vi "projector check.vi"() -> ()   [LabVIEW 2019]
uses:
  Setting Lib.lvlib
panel:
  out "Projector Status 26":bool
  out "Projector Status 30":bool
  out "Projector Status 29":bool
  out "Projector Status 27":bool
  out "Projector Status 28":bool
  out "error out 7":errorcluster
  in  "Threshold 26":dbl=0.01 format="%#_13g"
  in  "Threshold 30":dbl=0.01 format="%#_13g"
  in  "Threshold 29":dbl=0.01 format="%#_13g"
  in  "Threshold 27":dbl=0.01 format="%#_13g"
  in  "Threshold 28":dbl=0.01 format="%#_13g"
  out "error out 6":errorcluster
  out "error out 5":errorcluster
  out "error out 4":errorcluster
  out "error out 3":errorcluster
  out "error out 2":errorcluster
  out "error out":errorcluster
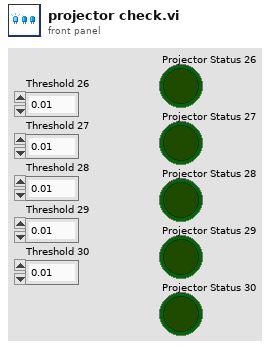
[diagram p1: front panel]
types:
  T1 = typedef "IMAQ Image.ctl" = refnum<image>
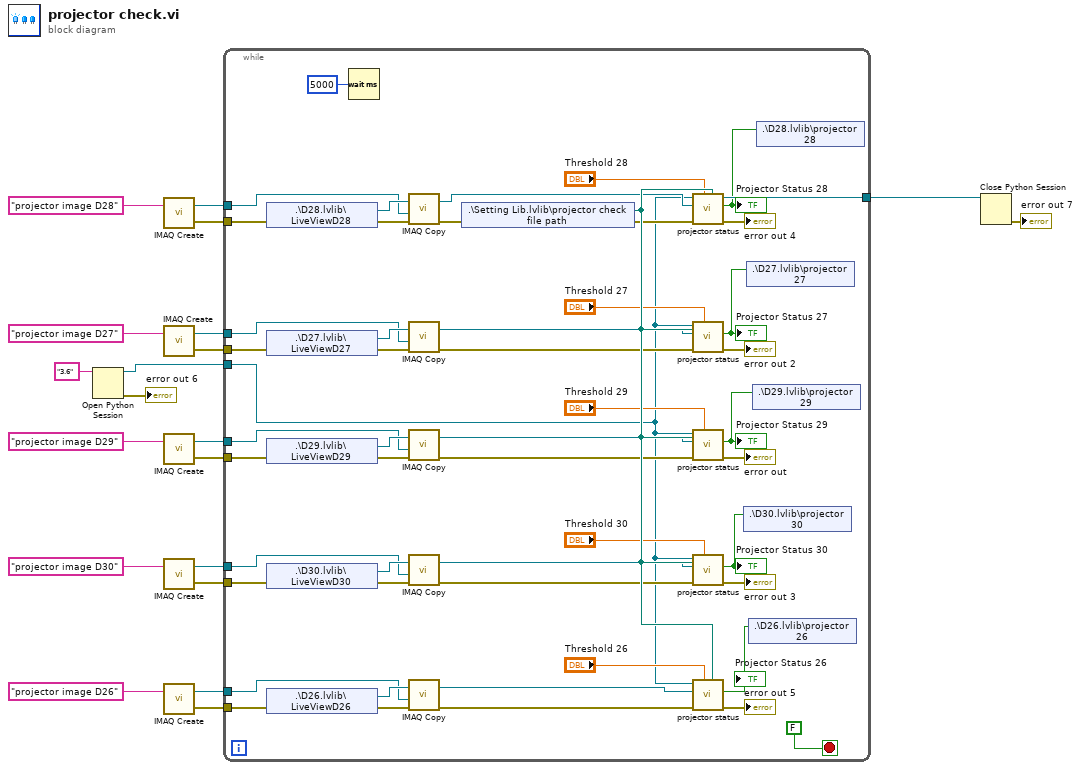
[diagram p0: block diagram]
diagram:
  n1 = Open Python Session(python version="3.6" ("Python version")) -> (session out=w3:refnum<k35>, error out=→"error out 6":errorcluster)  [unwired: 2 in]
  n2 = call "IMAQ Create"("Image Name"="projector image D28") -> ("New Image"=w11:T1, "error out"=w10:errorcluster)  [unwired: 4 in]
  n3 = call "IMAQ Create"("Image Name"="projector image D27") -> ("New Image"=w13:T1, "error out"=w12:errorcluster)  [unwired: 4 in]
  n4 = call "IMAQ Create"("Image Name"="projector image D29") -> ("New Image"=w9:T1, "error out"=w8:errorcluster)  [unwired: 4 in]
  n5 = call "IMAQ Create"("Image Name"="projector image D30") -> ("New Image"=w7:T1, "error out"=w6:errorcluster)  [unwired: 4 in]
  n6 = call "IMAQ Create"("Image Name"="projector image D26") -> ("New Image"=w15:T1, "error out"=w14:errorcluster)  [unwired: 4 in]
  n7 = while {
    tunnel: w15 -> [w66]
    tunnel: w14 -> [w65]
    tunnel: w13 -> [w58]
    tunnel: w12 -> [w57]
    tunnel: w11 -> [w52]
    tunnel: w10 -> [w51]
    tunnel: w9 -> [w45]
    tunnel: w8 -> [w44]
    tunnel: w7 -> [w38]
    tunnel: w6 -> [w37]
    tunnel: w3 -> [w28]
    tunnel: [w26] -> w2
    stop <- FALSE stop-if-true
    n8 = shared-variable ".\\D28.lvlib\\LiveViewD28"(error in=w51) -> (w54:refnum<image>, error out=w55:errorcluster)
    n9 = shared-variable ".\\D27.lvlib\\LiveViewD27"(error in=w57) -> (w62:refnum<image>, error out=w61:errorcluster)
    n10 = shared-variable ".\\D29.lvlib\\LiveViewD29"(error in=w44) -> (w49:refnum<image>, error out=w48:errorcluster)
    n11 = shared-variable ".\\D30.lvlib\\LiveViewD30"(error in=w37) -> (w41:refnum<image>, error out=w39:errorcluster)
    n12 = shared-variable ".\\D26.lvlib\\LiveViewD26"(error in=w65) -> (w70:refnum<image>, error out=w68:errorcluster)
    n13 = Wait (ms)(milliseconds to wait=u32 5000) -> ()  [unwired: 1 out]
    n14 = call "IMAQ Copy"("error in (no error)"=w55, "Image Dst"=w52, "Image Src"=w54) -> ("error out"=w35:errorcluster, "Image Dst Out"=w53:T1)  [unwired: 3 in]
    n15 = call "IMAQ Copy"("error in (no error)"=w61, "Image Dst"=w58, "Image Src"=w62) -> ("error out"=w60:errorcluster, "Image Dst Out"=w59:T1)  [unwired: 3 in]
    n16 = call "IMAQ Copy"("error in (no error)"=w48, "Image Dst"=w45, "Image Src"=w49) -> ("error out"=w47:errorcluster, "Image Dst Out"=w46:T1)  [unwired: 3 in]
    n17 = call "IMAQ Copy"("error in (no error)"=w39, "Image Dst"=w38, "Image Src"=w41) -> ("error out"=w42:errorcluster, "Image Dst Out"=w40:T1)  [unwired: 3 in]
    n18 = call "IMAQ Copy"("error in (no error)"=w68, "Image Dst"=w66, "Image Src"=w70) -> ("error out"=w67:errorcluster, "Image Dst Out"=w69:T1)  [unwired: 3 in]
    n19 = shared-variable ".\\Setting Lib.lvlib\\projector check file path"(error in=w35) -> (w63:path, error out=w34:errorcluster)
    n20 = call "projector status.vi"("module path"=w63, "Threshold"="Threshold 28", "error in"=w34, "Image IN"=w53, "session in"=w28) -> ("error out"=→"error out 4":errorcluster, "Projector Status"=w23:bool, "session out"=w26:refnum<k35>)  [unwired: 4 in]
    "Projector Status 28" <- w23
    n21 = call "projector status.vi"("module path"=w63, "Threshold"="Threshold 27", "error in"=w60, "Image IN"=w59, "session in"=w28) -> ("error out"=→"error out 2":errorcluster, "Projector Status"=w24:bool)  [unwired: 4 in, 1 out]
    "Projector Status 27" <- w24
    n22 = call "projector status.vi"("module path"=w63, "Threshold"="Threshold 29", "error in"=w47, "Image IN"=w46, "session in"=w28) -> ("error out"=→"error out":errorcluster, "Projector Status"=w22:bool)  [unwired: 4 in, 1 out]
    "Projector Status 29" <- w22
    n23 = call "projector status.vi"("module path"=w63, "Threshold"="Threshold 30", "error in"=w42, "Image IN"=w40, "session in"=w28) -> ("error out"=→"error out 3":errorcluster, "Projector Status"=w21:bool)  [unwired: 4 in, 1 out]
    "Projector Status 30" <- w21
    n24 = call "projector status.vi"("module path"=w63, "Threshold"="Threshold 26", "error in"=w67, "Image IN"=w69, "session in"=w28) -> ("error out"=→"error out 5":errorcluster, "Projector Status"=w25:bool)  [unwired: 4 in, 1 out]
    "Projector Status 26" <- w25
    n25 = shared-variable ".\\D30.lvlib\\projector 30"(w21) -> ()  [unwired: 1 in, 1 out]
    n26 = shared-variable ".\\D27.lvlib\\projector 27"(w24) -> ()  [unwired: 1 in, 1 out]
    n27 = shared-variable ".\\D26.lvlib\\projector 26"(w25) -> ()  [unwired: 1 in, 1 out]
    n28 = shared-variable ".\\D29.lvlib\\projector 29"(w22) -> ()  [unwired: 1 in, 1 out]
    n29 = shared-variable ".\\D28.lvlib\\projector 28"(w23) -> ()  [unwired: 1 in, 1 out]
  }
  n30 = Close Python Session(session in=w2) -> (11:→"error out 7":errorcluster)  [unwired: 1 in]
